vi "Create Stream.vi"(8 "error in (no error)":errorcluster, 10 "VISA resource name":refnum<visa-resource-name>, 11 "Serial Client in":refnum<class "Serial Client.lvclass">) -> (0 "error out":errorcluster, 3 "Serial Client out":refnum<class "Serial Client.lvclass">)   [LabVIEW 2020, in "Stream-Serial.lvlib" / "Serial Client.lvclass"]
uses:
  Serial Client.lvclass
  C:/Program Files (x86)/National Instruments/LabVIEW 2020/vi.lib/IlluminatedG/lv-stream/Endpoint/Endpoint.lvclass
  Serial Client.lvclass/Serial Client.ctl
  Serial Stream/Serial Stream.lvclass
  C:/Program Files (x86)/National Instruments/LabVIEW 2020/vi.lib/IlluminatedG/lv-stream/stream/Stream.lvclass
  <vilib>/IlluminatedG/lv-stream/Endpoint/Endpoint.lvclass
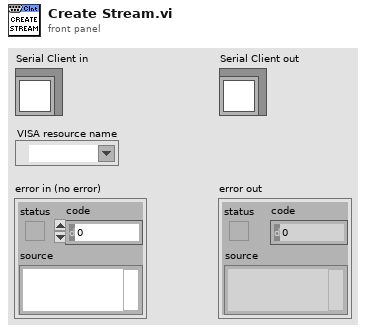
[diagram p1: front panel]
types:
  T1 = typedef "Stream-Serial.lvlib/Command Queue.ctl" = refnum<queue>
  T2 = typedef "Stream-Serial.lvlib/Serial Client.lvclass/Port Config.ctl" = cluster{"Baud (115200)":u32, "Data Bits (8)":u8, "Stop Bits (1)":T3, "Flow Control":T4, "Use LineTerm?":bool, "LineTerm (\\n)":string, "Timeout ms (10000)":i32, "Parity (None)":T5}
  T3 = typedef "Stream-Serial.lvlib/Serial Client.lvclass/Stop Bits.ctl" = u16
  T4 = typedef "Stream-Serial.lvlib/Serial Client.lvclass/Flow Control.ctl" = u16
  T5 = typedef "Stream-Serial.lvlib/Serial Client.lvclass/Parity.ctl" = enum16{"None", "Odd", "Even", "Mark", "Space"}
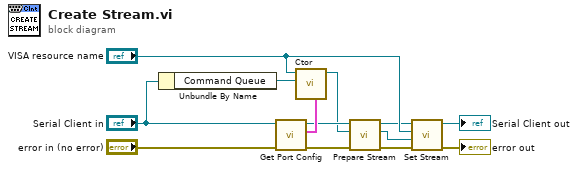
[diagram p0: block diagram]
diagram:
  n1 = Unbundle By Name("Serial Client in") -> ("Command Queue"=w13:T1)
  n2 = call "Get Port Config.vi"("error in (no error)"="error in (no error)", "Serial Client in"="Serial Client in") -> ("error out"=w6:errorcluster, "Port Config"=w12:T2, "Serial Client out"=w8:refnum<class "Serial Client.lvclass">)  [unwired: 7 in]
  n3 = call "Ctor.vi"("Port Config"=w12, "Command Queue"=w13, "VISA resource name"="VISA resource name") -> ("Serial Stream out"=w7:refnum<class "Serial Stream.lvclass">)  [unwired: 7 in, 1 out]
  n4 = call <vilib>:"Prepare Stream.vi"("error in (no error)"=w6, "Stream In"=w7, "Endpoint in"=w8) -> ("error out"=w5:errorcluster, "Stream"=w4:refnum<class "Serial Stream.lvclass">, "Endpoint out"=w3:refnum<class "Serial Client.lvclass">)  [unwired: 6 in]
  n5 = call "Set Stream.vi"("error in (no error)"=w5, "Stream"=w4, "VISA resource name"="VISA resource name", "Serial Client in"=w3) -> ("error out"=→"error out":errorcluster, "Serial Client out"=→"Serial Client out":refnum<class "Serial Client.lvclass">)  [unwired: 6 in]
